vi "servostay.vi"() -> ()   [LabVIEW 2017]
panel:
  out "stay":dbl
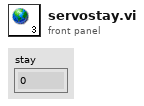
[diagram p1: front panel]
diagram:
